vi "Clamp_Example.vi"() -> ()   [LabVIEW 2019]
uses:
  <vilib>/Rock Robotics/WPI/ThirdParty/JAS_Junk/TrajLib/Trajectory_Library.lvlib
panel:
  out "Clamped\nOutput":dbl format="%14.3f"
  in  "High Limit":dbl=6.0
  in  "Input":dbl(slide)=10.0 scale=-100.0..100.0
  in  "Low Limit":dbl=1.0
  out "Clamped Vlue":cluster{"Input":dbl, "Result":dbl}(graph)
  out "Unclmaped\nInput":dbl=10.0 format="%14.3f"
  # "Analog  - Clamp - Example"
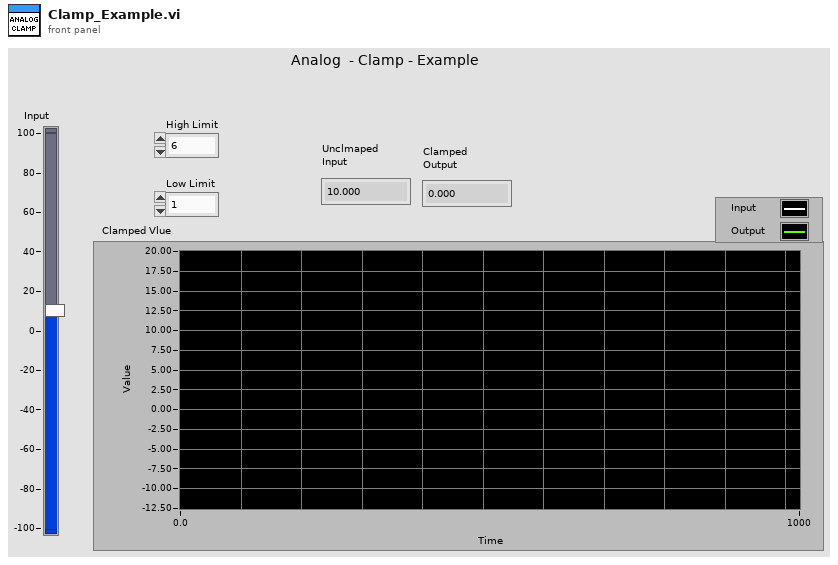
[diagram p1: front panel]
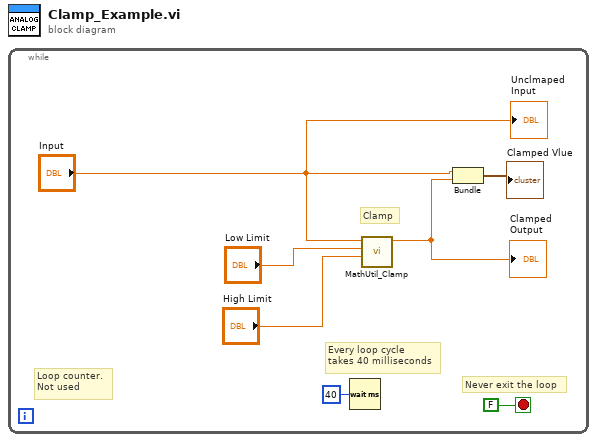
[diagram p0: block diagram]
diagram:
  n1 = while {
    stop <- FALSE stop-if-true
    # "Every loop cycle\ntakes 40 milliseconds"
    # "Clamp"
    # "Loop counter.\nNot used"
    # "Never exit the loop"
    n2 = Wait (ms)(milliseconds to wait=u32 40) -> ()  [unwired: 1 out]
    n3 = call <vilib>:"MathUtil_Clamp.vi"("High Limit"="High Limit", "Low Limit"="Low Limit", "Value"="Input") -> ("Result"=w4:dbl)  [unwired: 8 in]
    "Clamped\nOutput" <- w4
    n4 = Bundle("Input"="Input", "Result"=w4) -> (→"Clamped Vlue":cluster{"Input":dbl, "Result":dbl})  [unwired: 1 in]
    "Unclmaped\nInput" <- "Input"
  }
